vi "Search string in an Array LV2012 NI verified.vi"() -> ()   [LabVIEW 2023]
uses:
  <vilib>/regexp/Match Regular Expression.xnode
panel:
  in  "Ignore case":bool
  out "Error Out":errorcluster
  in  "Error In":errorcluster
  out "Index of array":i32
  out "Element":string
  in  "Array - String":string[](array[string])
  in  "Search For":string
  # "Overview:Use this VI to search the first element of a string array that contains a specific substring. \nRequirements: LabVIEW 2012\nInstructions:\n1. Insert an Array \n2. Select the string that you want to find\n3. Press Ignore case switch to do a case insensitive search"
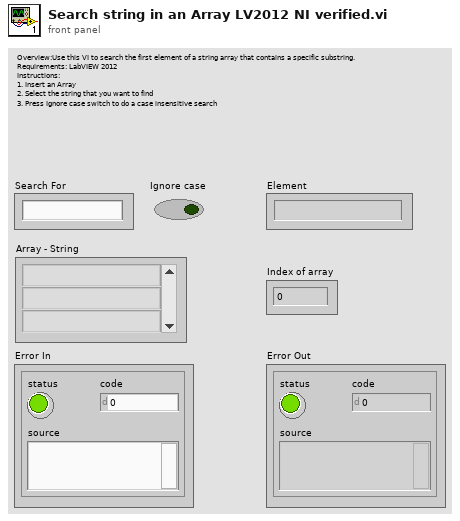
[diagram p1: front panel]
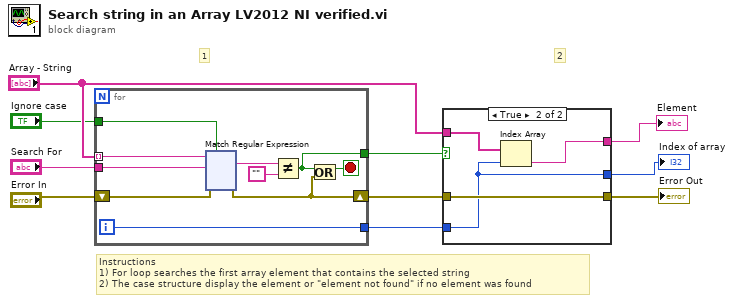
[diagram p0: block diagram]
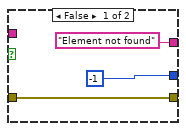
[diagram p2: hidden frame]
diagram:
  # "Instructions\n1) For loop searches the first array element that contains the selected string\n2) The case structure display the element or \"element not found\" if no element was found"
  # "2"
  # "1"
  n1 = for {
    tunnel: "Array - String" -> [w20] mode=indexing
    tunnel: [w17] -> w5
    tunnel: "Search For" -> [w18]
    shift-right: [w11] -> w3
    shift-left: "Error In" -> [w12]
    tunnel: [w15] -> w6
    tunnel: "Ignore case" -> [w13]
    i -> [w17]
    stop <- w14 stop-if-true
    n2 = xnode "Match Regular Expression"("input string"=w20, "regular expression"=w18, "error in"=w12, "ignore case? (F)"=w13) -> ("whole match"=w19:string, "error out"=w11:errorcluster)  [unwired: 2 in, 3 out]
    n3 = Not Equal?(x=w19, y="") -> (x != y?=w15:bool)
    n4 = Or(x=w15, y=w11) -> (x .or. y?=w14:bool)
  }
  n5 = case shown="True" w6 {
    tunnel: w5 -> [_ w141]
    tunnel: "Array - String" -> [_ w144]
    tunnel: ["Element not found" ("String") w143] -> w7
    tunnel: [-1 w141] -> w4
    tunnel: w3 -> [w138 w142]
    tunnel: [w138 w142] -> w2
    frame False {
    }
    frame True {
      n6 = Index Array(array=w144, index=w141) -> (element=w143:string)
    }
  }
  "Error Out" <- w2
  "Element" <- w7
  "Index of array" <- w4
